vi "Event Self.vi"(10 "Msg Strategy":refnum<class "Msg Strategy.lvclass">, 11 "Event jettl in":refnum<class "Event jettl.lvclass">) -> (3 "Event jettl out":refnum<class "Event jettl.lvclass">)   [LabVIEW 2021, in "jettl.lvlib" / "Event jettl.lvclass"]
uses:
  Event jettl.lvclass
  Msg Strategy/Msg Strategy/Msg Strategy.lvclass
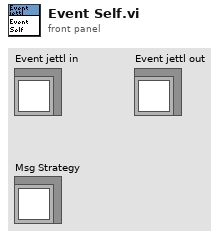
[diagram p1: front panel]
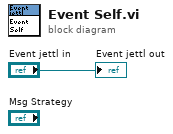
[diagram p0: block diagram]
diagram:
  "Event jettl out" <- "Event jettl in"
